vi "DSF.Engine.Memory.Pointer.Array.Allocate.vi"(8 "error in (no error)":errorcluster, 9 "count (1)":u64=1 format="%d elements", 10 "element size":u64 format="%d bytes", 11 "Array Pointer in":refnum<class "DSF.Engine.Memory.Pointer.Array.lvclass">) -> (0 "error out":errorcluster, 3 "Array Pointer out":refnum<class "DSF.Engine.Memory.Pointer.Array.lvclass">)   [LabVIEW 2016, in "DSF.Engine.lvlib" / "DSF.Engine.Memory.Pointer.Array.lvclass"]
uses:
  Memory.Pointer/DSF.Engine.Memory.Pointer.Array.lvclass
  C:/Git/Sourcetree/DSF/Source/Submodules/Memory Manager/Source/Classes/Pointer.Internal/Memory.Pointer.Internal.lvclass
  Memory.Pointer/DSF.Engine.Memory.Pointer.Array.lvclass/DSF.Engine.Memory.Pointer.Array.ctl
  Submodules/Memory Manager/Source/Classes/Pointer.Internal/Memory.Pointer.Internal.lvclass
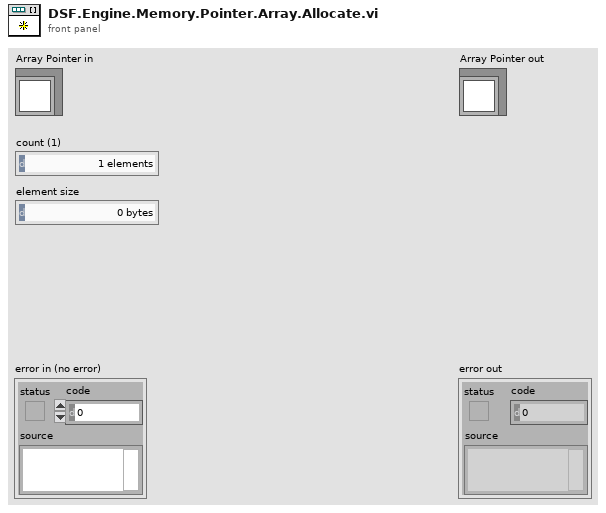
[diagram p1: front panel]
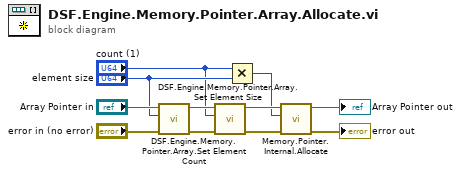
[diagram p0: block diagram]
diagram:
  n1 = call "DSF.Engine.Memory.Pointer.Array.Set Element Size.vi"("error in (no error)"="error in (no error)", "element size"="element size", "Array Pointer in"="Array Pointer in") -> ("error out"=w5:errorcluster, "Array Pointer out"=w6:refnum<class "DSF.Engine.Memory.Pointer.Array.lvclass">)  [unwired: 7 in]
  n2 = call "DSF.Engine.Memory.Pointer.Array.Set Element Count.vi"("error in (no error)"=w5, "element count"="count (1)", "Array Pointer in"=w6) -> ("error out"=w3:errorcluster, "Array Pointer out"=w4:refnum<class "DSF.Engine.Memory.Pointer.Array.lvclass">)  [unwired: 7 in]
  n3 = Multiply(x="count (1)", y="element size") -> (x*y=w2:u64)
  n4 = call "Memory.Pointer.Internal.Allocate.vi"("error in (no error)"=w3, "size"=w2, "pointer in"=w4) -> ("error out"=→"error out":errorcluster, "pointer out"=→"Array Pointer out":refnum<class "DSF.Engine.Memory.Pointer.Array.lvclass">)  [unwired: 7 in]
